vi "BoxCarFilter.vi"(9 "N Sigma (3)":dbl=3.0 min=0.0 format="%#_13g", 10 "Bin Size (7)":i32=7 min=1, 11 "Graph in":cluster{dbl[], dbl[]}) -> (2 "Window Size":dbl=4.0 format="%#_13g", 3 "Graph out":cluster{dbl[], dbl[]})   [LabVIEW 2019]
uses:
  <vilib>/Analysis/NI_AALBase.lvlib
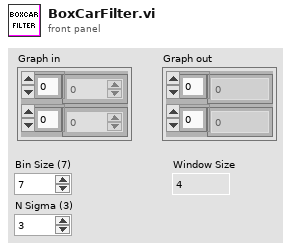
[diagram p1: front panel]
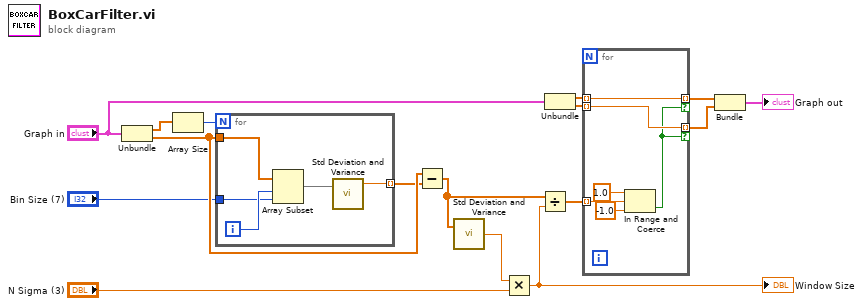
[diagram p0: block diagram]
diagram:
  n1 = Unbundle("Graph in") -> (w15:dbl[], w16:dbl[])
  n2 = Array Size(array=w15) -> (size(s)=w8:i32)
  n3 = for {
    N: w8 -> [_]
    tunnel: w16 -> [w21]
    tunnel: "Bin Size (7)" -> [w19]
    tunnel: [w17] -> w9 mode=indexing
    i -> [w20]
    n4 = Array Subset(array=w21, index=w20, length=w19) -> (w18:dbl[])
    n5 = call <vilib>:"Std Deviation and Variance.vi"("X"=w18) -> ("mean"=w17:dbl)  [unwired: 1 in, 2 out]
  }
  n6 = Subtract(x=w16, y=w9) -> (x-y=w11:dbl[])
  n7 = call <vilib>:"Std Deviation and Variance.vi"("X"=w11) -> ("standard deviation"=w12:dbl)  [unwired: 1 in, 2 out]
  n8 = Multiply(x=w12, y="N Sigma (3)") -> (x*y=w13:dbl)
  "Window Size" <- w13
  n9 = Divide(x=w11, y=w13) -> (x/y=w7:dbl[])
  n10 = Unbundle("Graph in") -> (w4:dbl[], w2:dbl[])
  n11 = for {
    tunnel: w4 -> [w24] mode=indexing
    tunnel: w2 -> [w23] mode=indexing
    tunnel: w7 -> [w27] mode=indexing
    tunnel: [w24] -> w6 mode=indexing if=w22
    tunnel: [w23] -> w5 mode=indexing if=w22
    n12 = In Range and Coerce(upper limit=1.0, x=w27, lower limit=-1.0 ("upper limit")) -> (In Range?=w22:bool)  [unwired: 1 out]
  }
  n13 = Bundle(w6, w5) -> (→"Graph out":cluster{dbl[], dbl[]})  [unwired: 1 in]
